vi "SysParamGetRef.vi"(0 "R Sense [Ohms] in":refnum<vi>, 1 "Op Amp Gain in":refnum<vi>, 2 "Temp High Th":refnum<vi>, 3 "RingCancelDelay":refnum<vi>, 4 "Vin High Th":refnum<vi>, 5 "Unit Add in":refnum<vi>, 6 "Temp Low Th":refnum<vi>, 7 "Vin Low Th":refnum<vi>, 8 "System Up Time in":refnum<vi>, 9 "Init":bool, 10 "System Total Time":refnum<vi>, 11 "Sys Tech.Data S":refnum<vi>, 12 "System General data":refnum<vi>) -> (15 "System General data out":refnum<vi>, 16 "Op Amp Gain out":refnum<vi>, 18 "System Total Time out":refnum<vi>, 19 "Sys Tech.Data S out":refnum<vi>, 20 "R Sense [Ohms] out":refnum<vi>, 21 "RingCancelDelay out":refnum<vi>, 22 "Temp High Th out":refnum<vi>, 23 "Vin High Th out":refnum<vi>, 24 "Vin Low Th out":refnum<vi>, 25 "Unit Add out":refnum<vi>, 26 "Temp Low Th out":refnum<vi>, 27 "System Up Time  out":refnum<vi>)   [LabVIEW 2017]
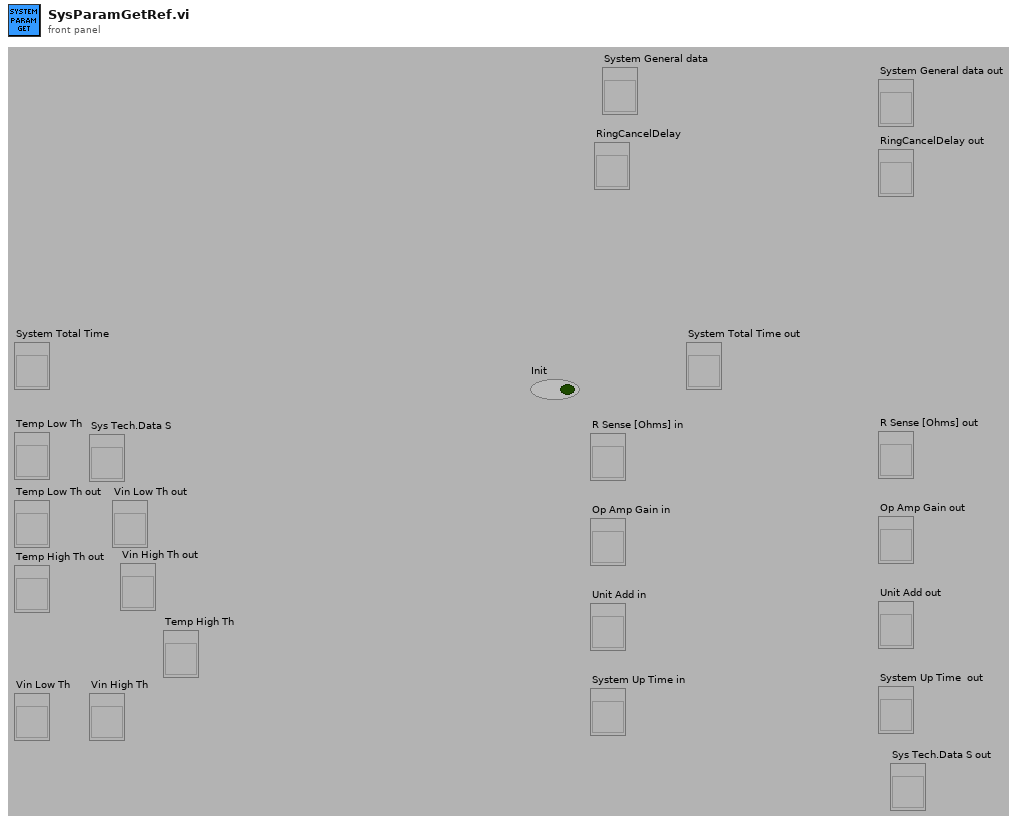
[diagram p1: front panel]
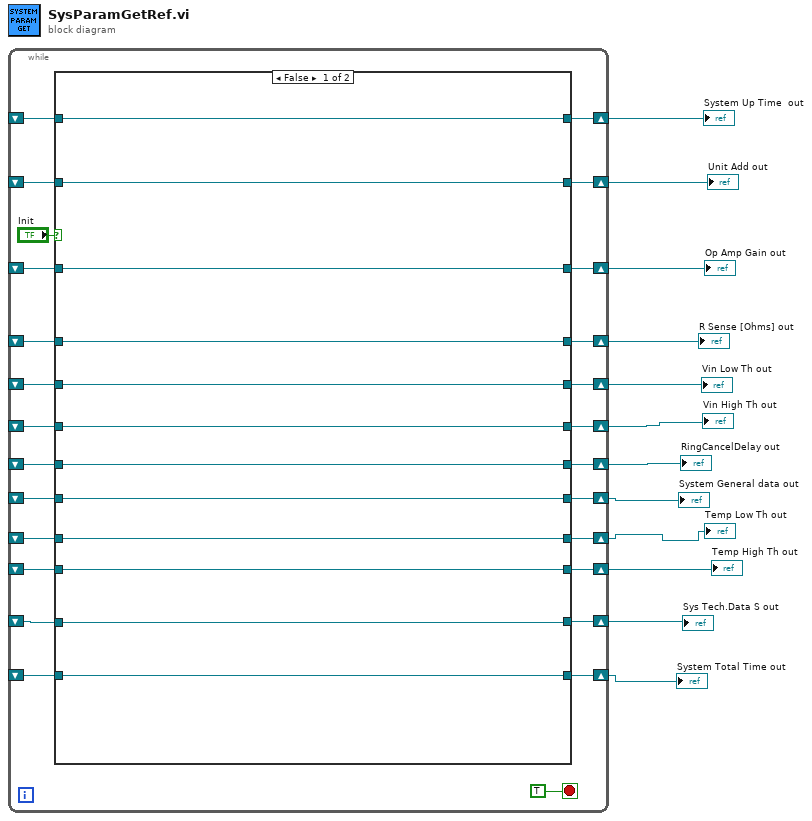
[diagram p0: block diagram]
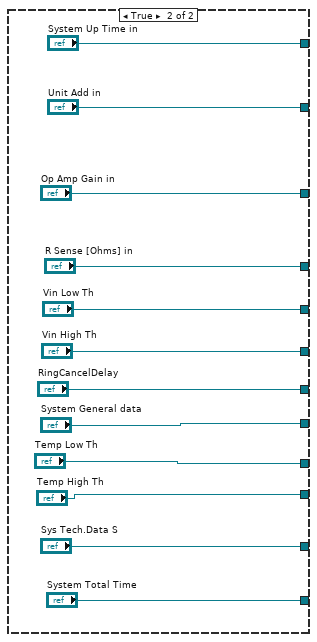
[diagram p2: hidden frame]
diagram:
  n1 = while {
    shift-right: [w36] -> w12
    shift-left: _ -> [w32]
    shift-right: [w35] -> w11
    shift-left: _ -> [w31]
    shift-right: [w34] -> w10
    shift-left: _ -> [w30]
    shift-right: [w33] -> w9
    shift-left: _ -> [w29]
    shift-right: [w28] -> w6
    shift-left: _ -> [w25]
    shift-right: [w27] -> w5
    shift-left: _ -> [w24]
    shift-right: [w26] -> w8
    shift-left: _ -> [w23]
    shift-right: [w22] -> w7
    shift-left: _ -> [w21]
    shift-right: [w19] -> w3
    shift-left: _ -> [w17]
    shift-right: [w20] -> w4
    shift-left: _ -> [w18]
    shift-right: [w16] -> w2
    shift-left: _ -> [w15]
    shift-right: [w14] -> w1
    shift-left: _ -> [w13]
    stop <- TRUE stop-if-true
    n2 = case shown="False" "Init" {
      tunnel: [w50 "System Up Time in"] -> w36
      tunnel: [w49 "Unit Add in"] -> w35
      tunnel: [w48 "Op Amp Gain in"] -> w34
      tunnel: [w47 "R Sense [Ohms] in"] -> w33
      tunnel: w32 -> [w50 _]
      tunnel: w31 -> [w49 _]
      tunnel: w30 -> [w48 _]
      tunnel: w29 -> [w47 _]
      tunnel: [w46 "Vin Low Th"] -> w28
      tunnel: [w45 "Vin High Th"] -> w27
      tunnel: [w44 "RingCancelDelay"] -> w26
      tunnel: w25 -> [w46 _]
      tunnel: w24 -> [w45 _]
      tunnel: w23 -> [w44 _]
      tunnel: [w43 "System General data"] -> w22
      tunnel: w21 -> [w43 _]
      tunnel: [w42 "Temp Low Th"] -> w20
      tunnel: [w41 "Temp High Th"] -> w19
      tunnel: w18 -> [w42 _]
      tunnel: w17 -> [w41 _]
      tunnel: [w40 "Sys Tech.Data S"] -> w16
      tunnel: w15 -> [w40 _]
      tunnel: [w39 "System Total Time"] -> w14
      tunnel: w13 -> [w39 _]
      frame False {
      }
      frame True {
      }
    }
  }
  "System Up Time  out" <- w12
  "Unit Add out" <- w11
  "Op Amp Gain out" <- w10
  "R Sense [Ohms] out" <- w9
  "RingCancelDelay out" <- w8
  "System General data out" <- w7
  "Vin Low Th out" <- w6
  "Vin High Th out" <- w5
  "Temp Low Th out" <- w4
  "Temp High Th out" <- w3
  "Sys Tech.Data S out" <- w2
  "System Total Time out" <- w1
